vi "WSP2_PartNumberRef.vi"(0 "SerialNumber":string) -> (1 "AssemblyPartNumber":string, 2 "error out":errorcluster)   [LabVIEW 2023]
uses:
  C:/Elatch-Bench-Programming/WSConnector/WSConnector.dll
  WSConnector/WSConnector.dll
panel:
  out "Cimp_AssemblyPartNumber":string
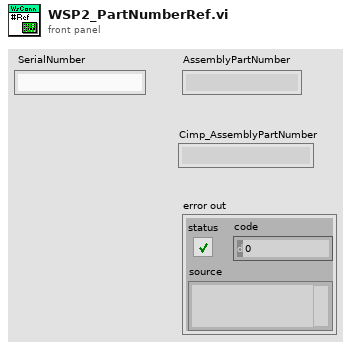
[diagram p1: front panel]
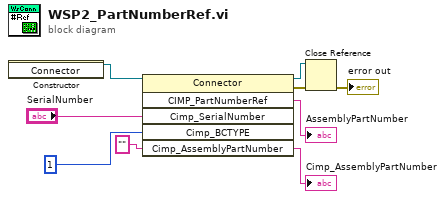
[diagram p0: block diagram]
diagram:
  n1 = constructor class="Connector"() -> (reference out=w9:refnum<k24>)  [unwired: 3 in, 2 out]
  n2 = invoke class="Connector" method="CIMP_PartNumberRef"(reference=w9, "Cimp_SerialNumber"="SerialNumber", "Cimp_BCTYPE"=1, "Cimp_AssemblyPartNumber"="") -> (reference out=w2:refnum<k24>, error out=w3:errorcluster, "CIMP_PartNumberRef"=→"AssemblyPartNumber":string, "Cimp_AssemblyPartNumber"=→"Cimp_AssemblyPartNumber":string)  [unwired: 2 in, 2 out]
  n3 = Close Reference(reference=w2, error in (no error)=w3) -> (error out=→"error out":errorcluster)
